vi "Get channels list.vi"(8 "error in (no error)":errorcluster, 11 "ActiveDev":tag="Dev4") -> (0 "error out":errorcluster, 3 "Channel list":tag[][](array[tag]))   [LabVIEW 2025]
uses:
  <resource>/objmgr/daqmx.rc
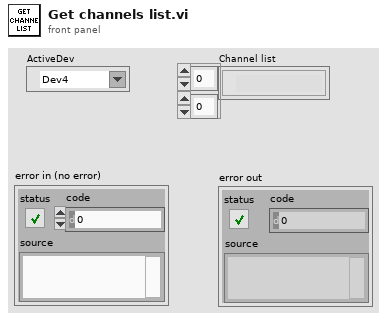
[diagram p1: front panel]
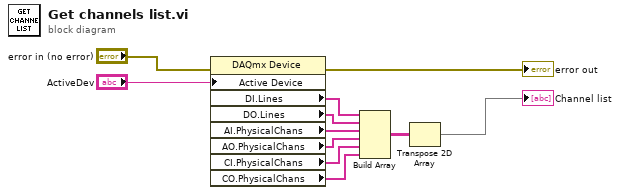
[diagram p0: block diagram]
diagram:
  n1 = property class="DAQmx Device"(error in="error in (no error)", "Active Device"="ActiveDev") -> (error out=→"error out":errorcluster, "DI.Lines"=w3:tag[], "DO.Lines"=w4:tag[], "AI.PhysicalChans"=w5:tag[], "AO.PhysicalChans"=w6:tag[], "CI.PhysicalChans"=w7:tag[], "CO.PhysicalChans"=w8:tag[])  [unwired: 1 in, 1 out]
  n2 = Build Array(w3, w4, w5, w6, w7, w8) -> (w9:tag[][])
  n3 = Transpose 2D Array(2D array=w9) -> (transposed array=→"Channel list":tag[][])
